vi "Get Valid Properties.vi"(8 "error in (no error)":errorcluster, 11 "Pulse Train in":refnum<class "Pulse Train.lvclass">) -> (0 "error out":errorcluster, 2 "Properties":string[](array[string]), 3 "Pulse Train out":refnum<class "Pulse Train.lvclass">)   [LabVIEW 2020, in "Pulse Train.lvclass"]
uses:
  Pulse Train.lvclass
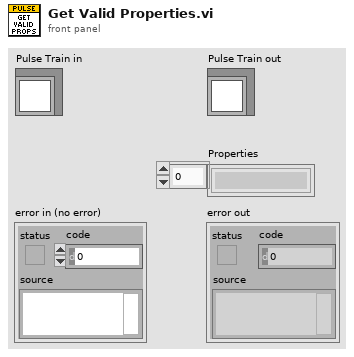
[diagram p1: front panel]
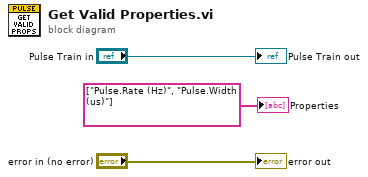
[diagram p0: block diagram]
diagram:
  "error out" <- "error in (no error)"
  "Pulse Train out" <- "Pulse Train in"
  "Properties" <- string[] ["Pulse.Rate (Hz)", "Pulse.Width (us)"] ("Properties")
